vi "Connect Channel Command.vi"(8 "error in (no error)":errorcluster, 10 "Channel Connection Data":T1 {"Connection Data" format="%x"}, 11 "CIFChannelMng in":refnum<class "CIFChannelMng.lvclass">) -> (0 "error out":errorcluster, 3 "CIFChannelMng out":refnum<class "CIFChannelMng.lvclass">)   [LabVIEW 2021, in "CIFChannelMng.lvclass"]
uses:
  CIFChannelMng.lvclass
  OOB/OOB_Rx/Typedef/Channel Connection Data.ctl
  CIFChannelMng.lvclass/CIFChannelMng.ctl
  <vilib>/CIF Foundation/CIF Out of Band Commands/CIFOutOfBand.lvclass/CIFOutOfBand.ctl
  <vilib>/CIF Foundation/CIF Out of Band Commands/Accessors/Read Local OOB Data.vi
  <vilib>/CIF Foundation/CIF Out of Band Commands/Queue Command.vi
  <vilib>/CIF Foundation/CIF Out of Band Commands/Utilities/Command to Bitwise Command.vi
  OOB/OOB_Rx/ChanMngOOB_Rx.lvclass
  C:/Program Files/National Instruments/LabVIEW 2021/vi.lib/CIF Foundation/CIF Out of Band Commands/CIFOutOfBand.lvclass
  <vilib>/CIF Foundation/CIF Out of Band Commands/CIFOutOfBand.lvclass
  D:/dev/CIF-LVCore/src/Channels/CIFChannelMng/OOB/OOB_Rx/ChanMngOOB_Rx.lvclass
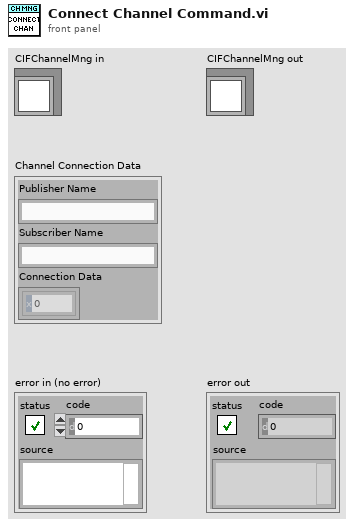
[diagram p1: front panel]
types:
  T1 = typedef "ChanMngOOB_Rx.lvclass/Channel Connection Data.ctl" = cluster{"Publisher Name":string, "Subscriber Name":string, "Connection Data":u8[]}
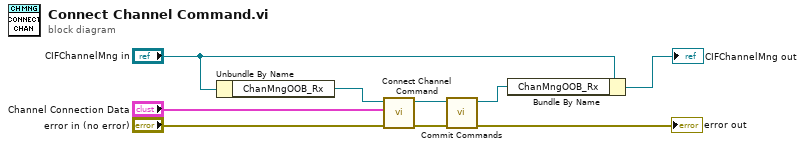
[diagram p0: block diagram]
diagram:
  n1 = Unbundle By Name("CIFChannelMng in") -> ("ChanMngOOB_Rx"=w6:refnum<class "ChanMngOOB_Rx.lvclass">)
  n2 = call "Connect Channel Command.vi"("error in"="error in (no error)", "Channel Connection Data"="Channel Connection Data", "ChanMngOOB_Rx in"=w6) -> ("error out"=w3:errorcluster, "ChanMngOOB_Rx out"=w4:refnum<class "ChanMngOOB_Rx.lvclass">)  [unwired: 7 in]
  n3 = call <vilib>:"Commit Commands.vi"("error in"=w3, "OOB in"=w4) -> ("error out"=→"error out":errorcluster, "OOB out"=w2:refnum<class "ChanMngOOB_Rx.lvclass">)  [unwired: 8 in]
  n4 = Bundle By Name(cluster="CIFChannelMng in", "ChanMngOOB_Rx"=w2) -> (→"CIFChannelMng out":refnum<class "CIFChannelMng.lvclass">)
